vi "Sub_DetailString.vi"(6 "Enum":T1(ring), 7 "Tabelle IN 2":refnum<vi>, 10 "String IN":string, 11 "Tabelle IN":string[][](table)) -> (2 "String OUT":string, 3 "Tabelle OUT":string[][](array[string]))   [LabVIEW 2015, in "Sprachverwaltung.lvlib" / "Bildzuordnung.lvlib"]
uses:
  Bildzuordnung.lvlib
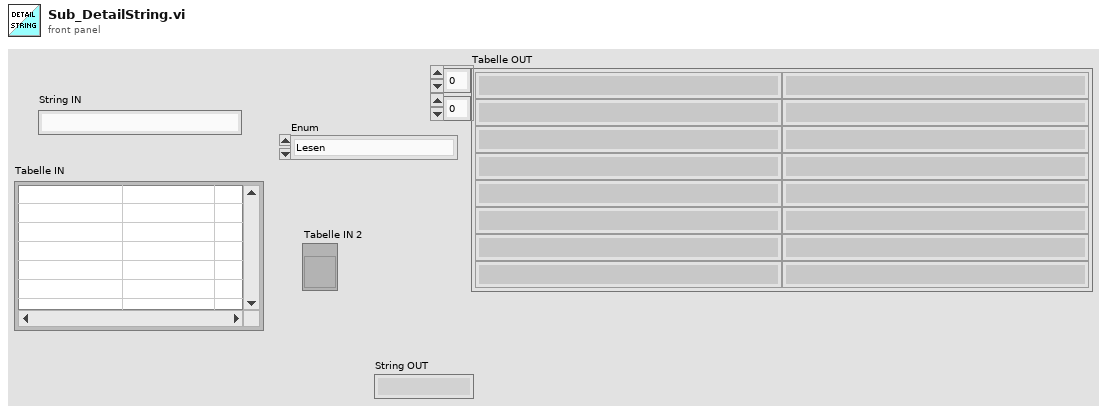
[diagram p1: front panel]
types:
  T1 = enum16{"Lesen", "String beschreiben", "Tabelle beschreiben"}
  T2 = typedef "LVRowAndColumnTypeDef.ctl" = cluster{"Row":i32, "Column":i32}
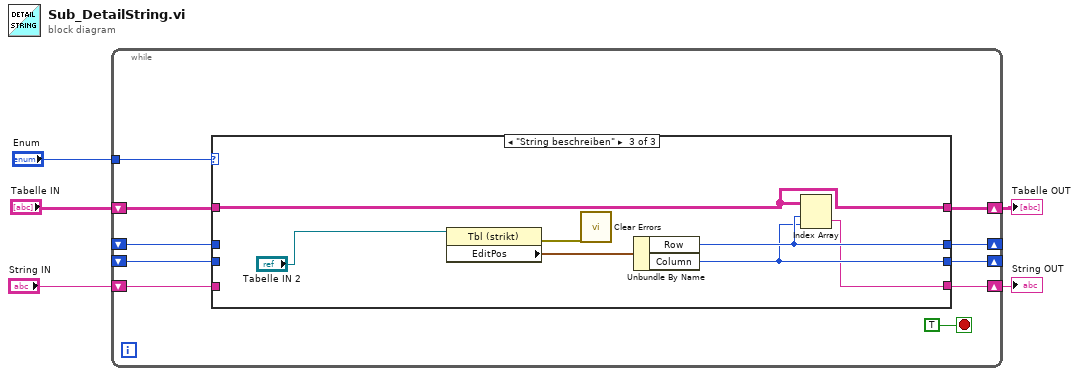
[diagram p0: block diagram]
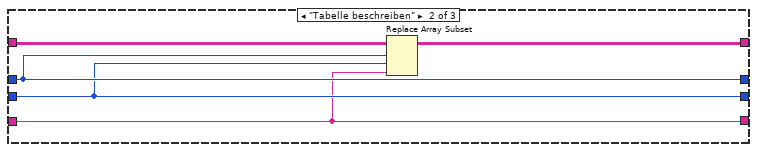
[diagram p3: hidden frame]
diagram:
  n1 = while {
    shift-right: [w10] -> w3
    shift-left: "Tabelle IN" -> [w15]
    shift-right: [w14] -> _
    shift-left: _ -> [w9]
    shift-right: [w13] -> _
    shift-left: _ -> [w8]
    tunnel: "Enum" -> [w11]
    shift-right: [w6] -> w1
    shift-left: "String IN" -> [w7]
    stop <- TRUE stop-if-true
    n2 = case shown="\"String beschreiben\"" w11 {
      tunnel: w15 -> [w19 w24 w28]
      tunnel: [w18 w22 w31] -> w14
      tunnel: [w17 w21 w30] -> w13
      tunnel: [w19 w23 w28] -> w10
      tunnel: w9 -> [w18 w22 _]
      tunnel: w8 -> [w17 w21 _]
      tunnel: w7 -> [w16 w20 _]
      tunnel: [w16 w20 w26] -> w6
      frame "Lesen", Default {
      }
      frame "Tabelle beschreiben" {
        n3 = Replace Array Subset(array=w24, new element=w20, index (row)=w22, index (col)=w21) -> (w23:string[][])
      }
      frame "String beschreiben" {
        n4 = property class="Tbl (strikt)"(reference="Tabelle IN 2") -> (error out=w27:errorcluster, "EditPos"=w29:T2)  [unwired: 1 in, 1 out]
        n5 = call <vilib>:"Clear Errors.vi"("error in (no error)"=w27) -> ()  [unwired: 5 in, 2 out]
        n6 = Unbundle By Name(w29) -> ("Row"=w31:i32, "Column"=w30:i32)
        n7 = Index Array(array=w28, index (row)=w31, index (col)=w30) -> (element=w26:string)
      }
    }
  }
  "Tabelle OUT" <- w3
  "String OUT" <- w1
